vi "AudioEffects.vi"() -> ()   [LabVIEW 2012]
panel:
  in  "?":bool
  in  "Boolean":bool
  out "Path at this Stage":path
  in  "Change Pitch?":bool
  out "Path at this Stage":path
  in  "Change Length?":bool
  in  "Speed":dbl
  out "Path at this Stage":path
  out "Path at this Stage":path
  out "Path at this Stage":path
  in  "Threshold":dbl(slide) scale=0.0..1.0
  in  "Add Distortion?":bool
  in  "Delay ms:":i32=5000
  in  "Magnitude":dbl=0.5
  in  "Add Echo?":bool
  in  "Recording Length (s)":i32=5
  in  "Output File":string
  in  "Output Directory":path
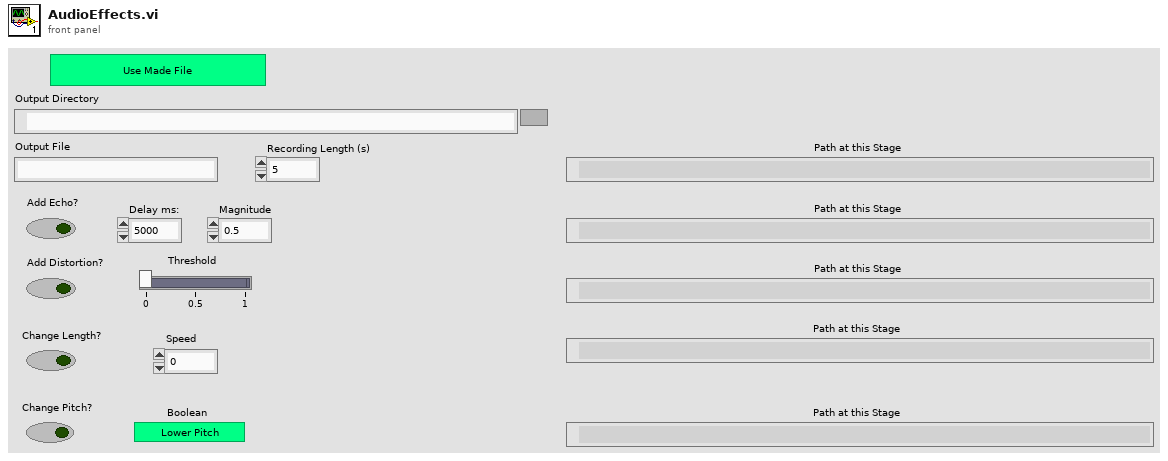
[diagram p1: front panel]
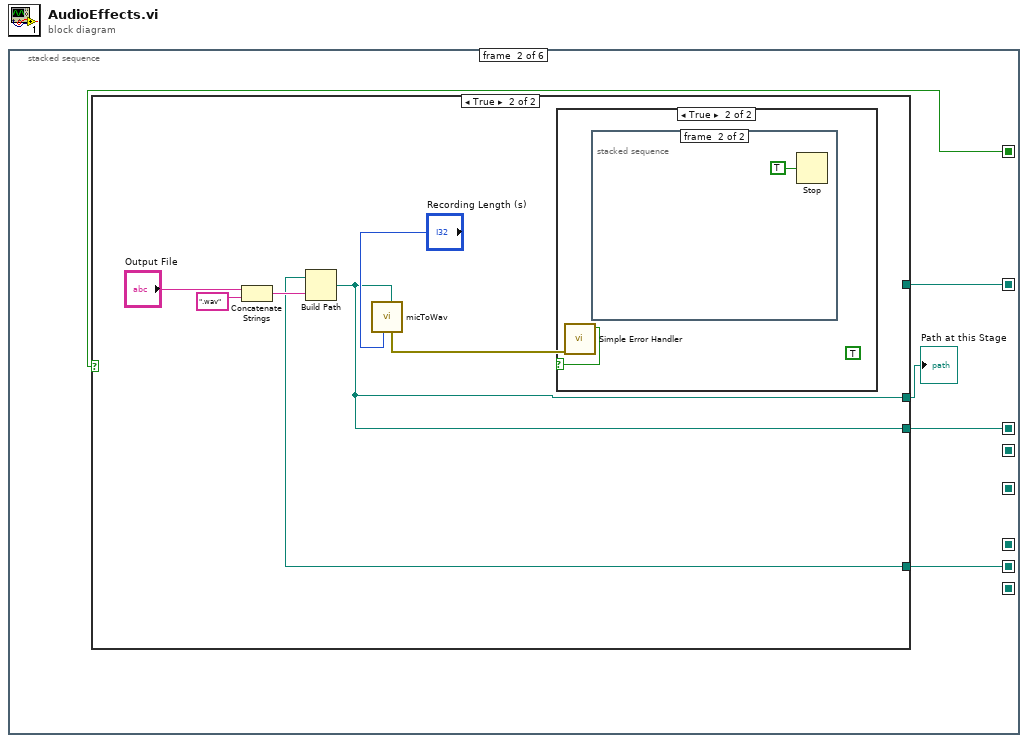
[diagram p0: block diagram]
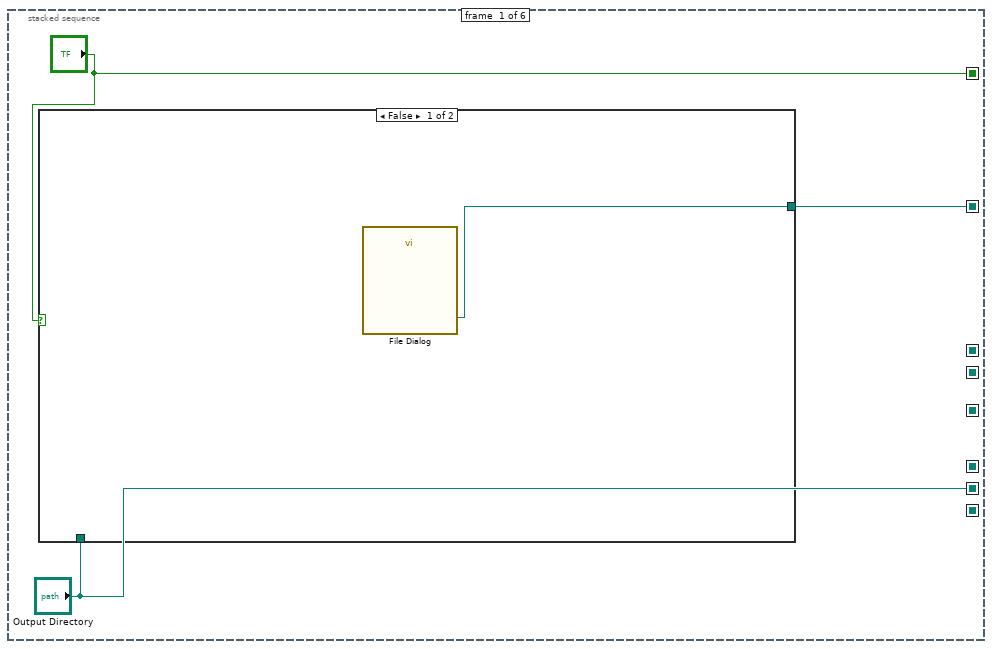
[diagram p2: hidden frame]
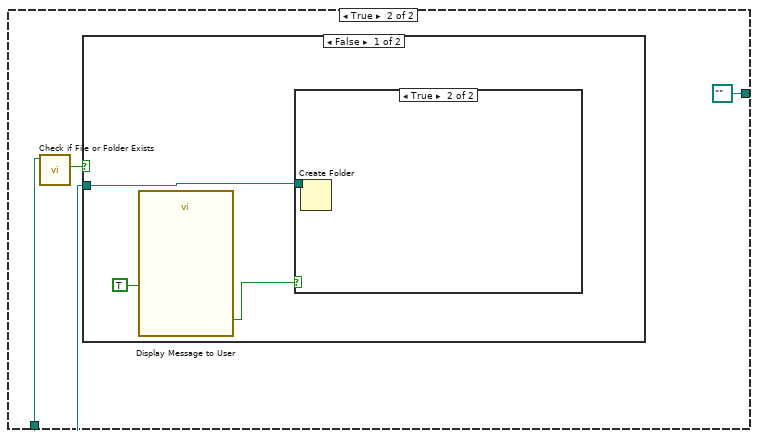
[diagram p3: hidden frame]
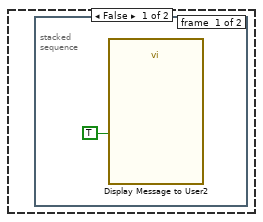
[diagram p4: hidden frame]
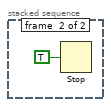
[diagram p5: hidden frame]
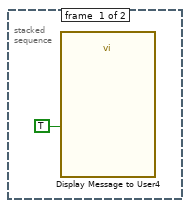
[diagram p9: hidden frame]
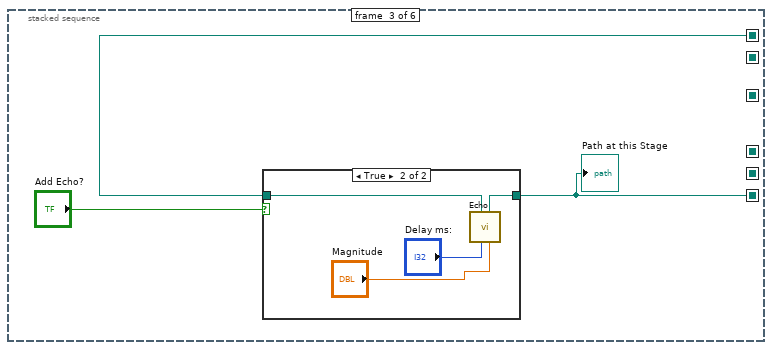
[diagram p10: hidden frame]
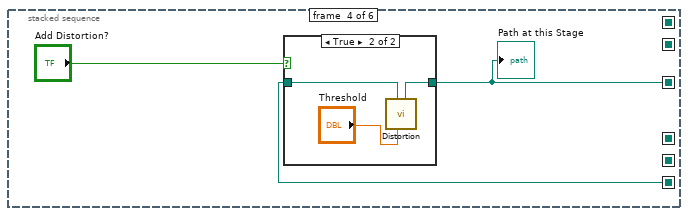
[diagram p12: hidden frame]
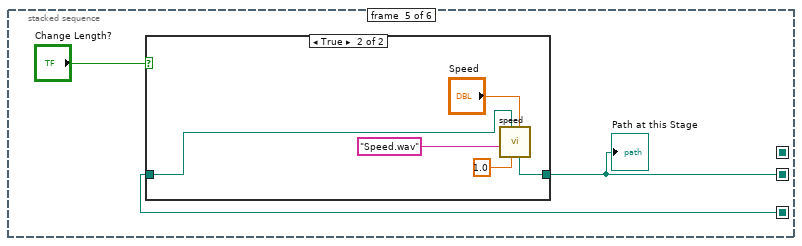
[diagram p14: hidden frame]
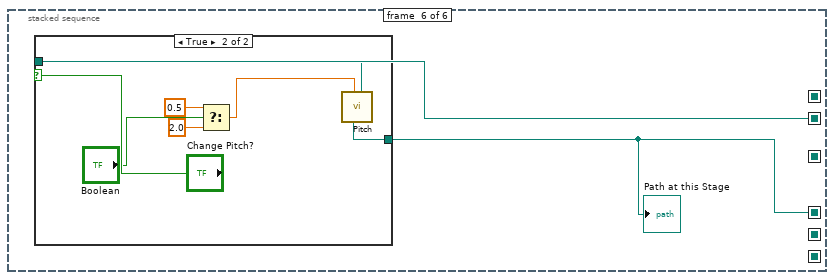
[diagram p16: hidden frame]
diagram:
  n1 = stacked-sequence {
    seq-local: ["Output Directory" _ _ _ _ _] -> [_ w18 _ _ _ _]
    seq-local: [_ w17 _ _ _ _] -> [_ _ w32 _ _ _]
    seq-local: [_ _ w31 _ _ _] -> [_ _ _ w40 _ _]
    seq-local: [_ _ _ w39 _ _] -> [_ _ _ _ w47 _]
    seq-local: [_ _ _ _ w45 _] -> [_ _ _ _ _ w55]
    seq-local: [_ _ _ _ _ w54] -> [_ _ _ _ _ _]
    seq-local: [w2 _ _ _ _ _] -> [_ w15 _ _ _ _]
    seq-local: ["?" _ _ _ _ _] -> [_ w16 _ _ _ _]
    frame #0 {
      n2 = case shown="False" "?" {
        tunnel: "Output Directory" -> [_ w6]
        tunnel: [w4 path "" ("selected path")] -> w2
        frame False {
          n3 = call "File Dialog"() -> ("selected path"=w4:path)  [unwired: 12 in, 3 out]
        }
        frame True {
          n4 = call <vilib>:"Check if File or Folder Exists.vi"("path"=w6) -> ("file or folder exists?"=w7:bool)  [unwired: 8 in, 2 out]
          n5 = case shown="False" w7 {
            tunnel: w6 -> [w8 _]
            frame False {
              n6 = call "Display Message to User"("Enable"=TRUE) -> ("OK"=w10:bool)  [unwired: 9 in, 1 out]
              n7 = case shown="True" w10 {
                tunnel: w8 -> [_ w13]
                frame False {
                  n8 = stacked-sequence {
                    frame #0 {
                      n9 = call "Display Message to User2"("Enable"=TRUE) -> ()  [unwired: 9 in, 2 out]
                    }
                    frame #1 {
                      n10 = Stop(stop? (T)=TRUE) -> ()
                    }
                  }
                }
                frame True {
                  n11 = Create Folder(path (use dialog)=w13) -> ()  [unwired: 2 in, 3 out]
                }
              }
            }
            frame True {
            }
          }
        }
      }
    }
    frame #1 {
      n12 = case shown="True" w16 {
        tunnel: w18 -> [_ w24]
        tunnel: [w19 w20] -> w17
        tunnel: w15 -> [w19 _]
        tunnel: [w19 w20] -> w14
        frame False {
        }
        frame True {
          n13 = Concatenate Strings("Output File", ".wav") -> (w25:string)
          n14 = Build Path(base path=w24, name or relative path=w25) -> (appended path=w20:path)
          n15 = call "micToWav.vi"("filename"=w20, "Sample Length (s)"="Recording Length (s)") -> ("error out"=w23:errorcluster)  [unwired: 9 in]
          n16 = call <vilib>:"Simple Error Handler.vi"("error in (no error)"=w23) -> ("error?"=w22:bool)  [unwired: 4 in, 4 out]
          n17 = case shown="True" w22 {
            frame False {
            }
            frame True {
              (unwired) TRUE ("Enable")
              n18 = stacked-sequence {
                frame #0 {
                  n19 = call "Display Message to User4"("Enable"=TRUE) -> ()  [unwired: 9 in, 2 out]
                }
                frame #1 {
                  n20 = Stop(stop? (T)=TRUE) -> ()
                }
              }
            }
          }
        }
      }
      "Path at this Stage" <- w14
    }
    frame #2 {
      n21 = case shown="True" "Add Echo?" {
        tunnel: w32 -> [w33 w35]
        tunnel: [w33 w34] -> w31
        frame False {
        }
        frame True {
          n22 = call "Echo.vi"("Magnitude"="Magnitude", "Delay ms:"="Delay ms:", "Input"=w35) -> ("output"=w34:path)  [unwired: 8 in]
        }
      }
      "Path at this Stage" <- w31
    }
    frame #3 {
      n23 = case shown="True" "Add Distortion?" {
        tunnel: w40 -> [w41 w44]
        tunnel: [w41 w43] -> w39
        frame False {
        }
        frame True {
          n24 = call "Distortion.vi"("Threshold"="Threshold", "Input"=w44) -> ("Output"=w43:path)  [unwired: 9 in]
        }
      }
      "Path at this Stage" <- w39
    }
    frame #4 {
      n25 = case shown="True" "Change Length?" {
        tunnel: w47 -> [w48 w53]
        tunnel: [w48 w51] -> w45
        frame False {
        }
        frame True {
          n26 = call "speed.vi"("speed"="Speed", "dt Scaling"=1.0, "input"=w53, "replacementString"="Speed.wav") -> ("output"=w51:path)  [unwired: 7 in]
        }
      }
      "Path at this Stage" <- w45
    }
    frame #5 {
      n27 = case shown="True" "Change Pitch?" {
        tunnel: w55 -> [w57 w63]
        tunnel: [w57 w62] -> w54
        frame False {
        }
        frame True {
          n28 = Select(t=0.5, s="Boolean", f=2.0) -> (s? t:f=w58:dbl)
          n29 = call "Pitch.vi"("input"=w63, "Pitch"=w58) -> ("output"=w62:path)  [unwired: 9 in]
        }
      }
      "Path at this Stage" <- w54
    }
  }
